vi "Length_7.vi"() -> ()   [LabVIEW 2020]
uses:
  Support/Controls/Cmd_Mouse Popup.ctl
  Support/Controls/Clst_Initialize Input.ctl
  Support/Controls/Cmd_Var Data IO.ctl
  Variables/Global_Cal Info.vi
  Variables/Global_Cal STD.vi
  Support/Public/Polymorph/Data Class_2D Str.vi
panel:
  out "STD set":string[][](table) caption="○ 기준기 조합 (값)"
  in  "기준기 설정":string(combo)
  in  "Measured 3":string[][](table)
  in  "Measured 2":string[][](table) caption="평행도 (μm)"
  out "최소범위":string
  out "단위":string
  out "최대범위":string
  in  "Spec 변경":bool
  in  "Random":bool
  out "Spec":string[][](table)
  out "제목":string
  out "에러 출력":errorcluster
  out "Condition":string[][](table) caption="2. 직선성 시험"
  in  "Measured":string[][](table) caption="지시편차 (μm)"
  out "Load?":bool
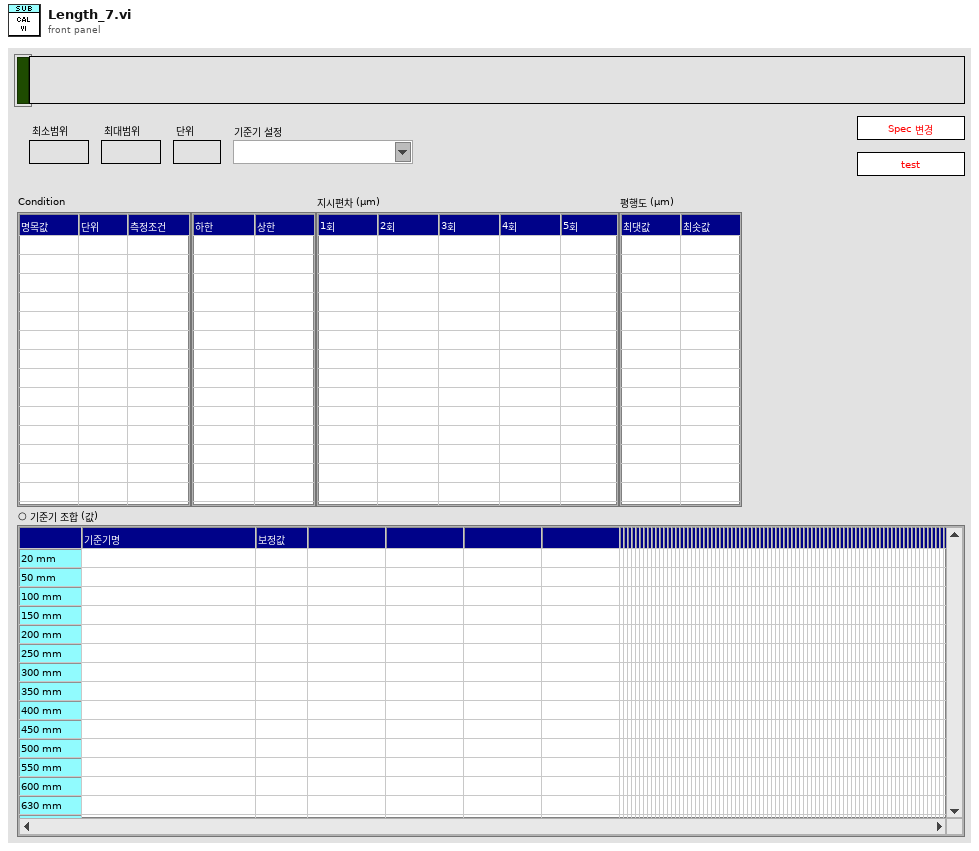
[diagram p1: front panel]
types:
  T1 = typedef "Cmd_Mouse Popup.ctl" = enum16{"활성화", "메뉴선택"}
  T2 = cluster{"Shift":bool, "Ctrl":bool, "Alt":bool, "Cmd":bool, "Opt":bool}
  T3 = typedef "Clst_Initialize Input.ctl" = cluster{"Initialize 1":cluster{"Condition":refnum<vi>[], "Spec":refnum<vi>[], "Measured":refnum<vi>[], "Resolution":refnum<vi>[], "Func_ext":string, "제목":refnum<vi>, "Measured_ADJ":refnum<vi>[]}, "Initialize 2":cluster{"문자열":refnum<vi>[], "콤보박스":refnum<vi>[], "링":refnum<vi>[], "열거형":refnum<vi>[], "테이블":refnum<vi>[], "여러열":refnum<vi>[], "디지털(DBL)":refnum<vi>[], "3D string":refnum<vi>[], "ctrl":refnum<vi>[], "boolean":refnum<vi>[]}}
  T4 = typedef "Cmd_Var Data IO.ctl" = enum16{"Condition", "Condition Default", "Condition_Temp", "Resolution", "Resolution Default", "Resolution Old", "Spec", "Spec Default", "Spec Old", "Spec Temp", "Result", "Result2", "Result3", "Result_Temp", "Result_ADJ", "Result_ADJ2", "STD1", "STD2", "STD3", "STD4", "STD5", "STD Temp", "CMC", "CMC Default"}
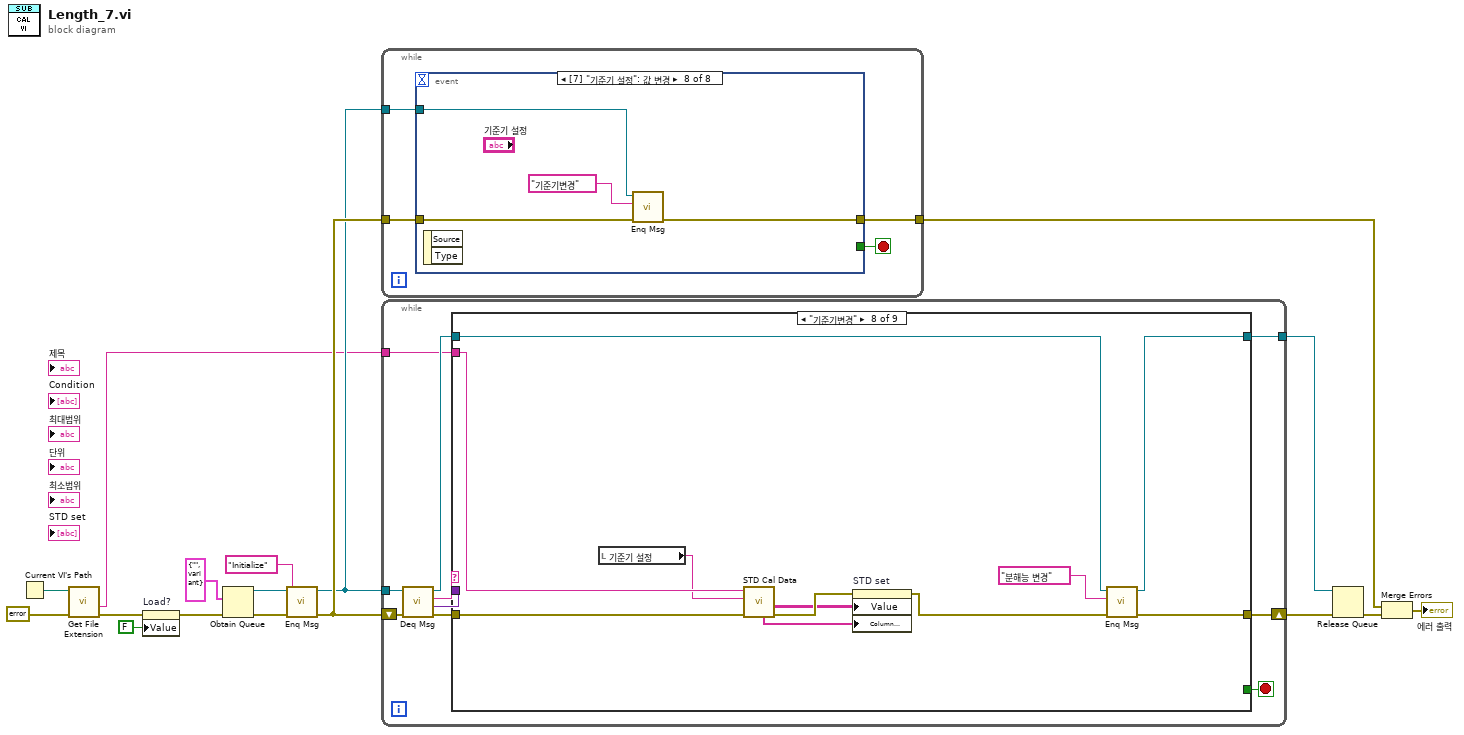
[diagram p0: block diagram]
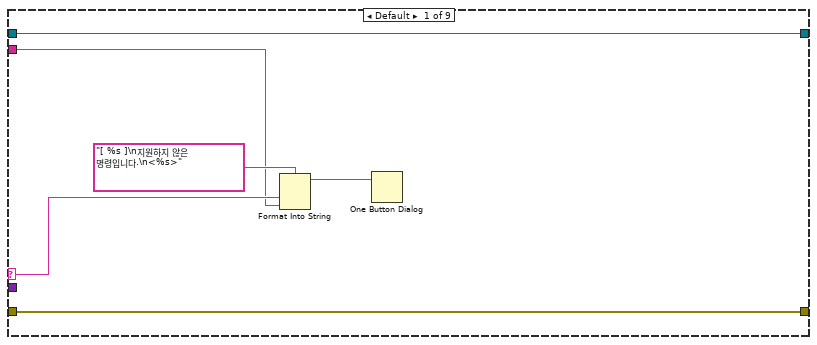
[diagram p2: hidden frame]
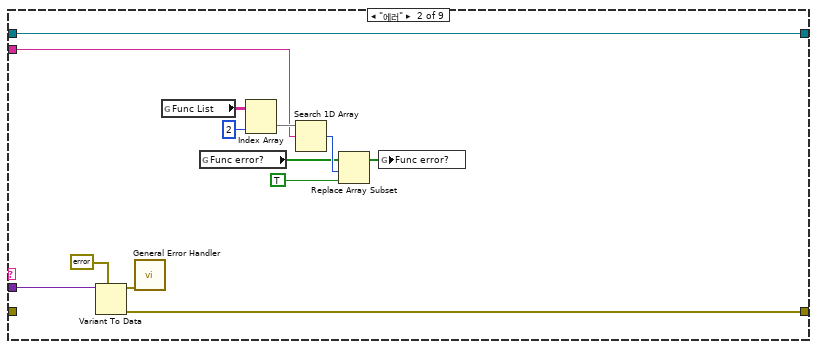
[diagram p3: hidden frame]
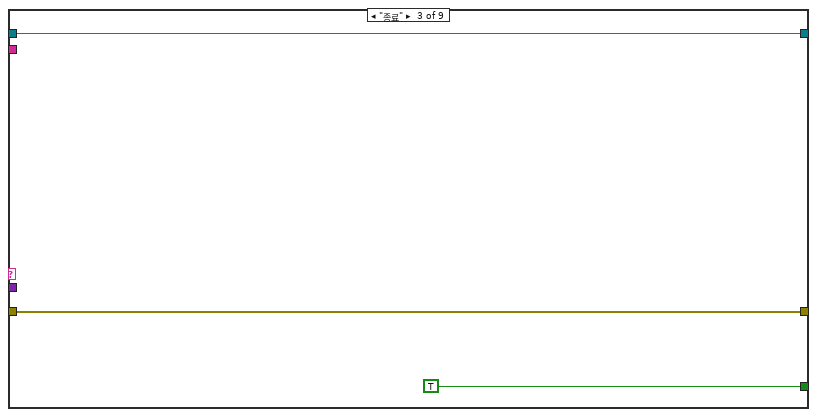
[diagram p4: hidden frame]
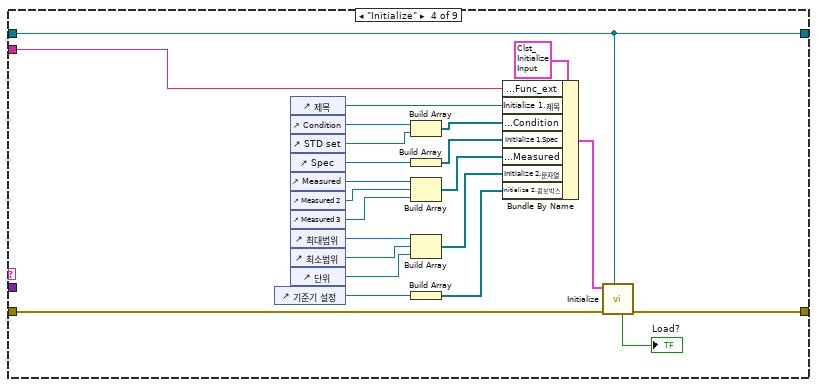
[diagram p5: hidden frame]
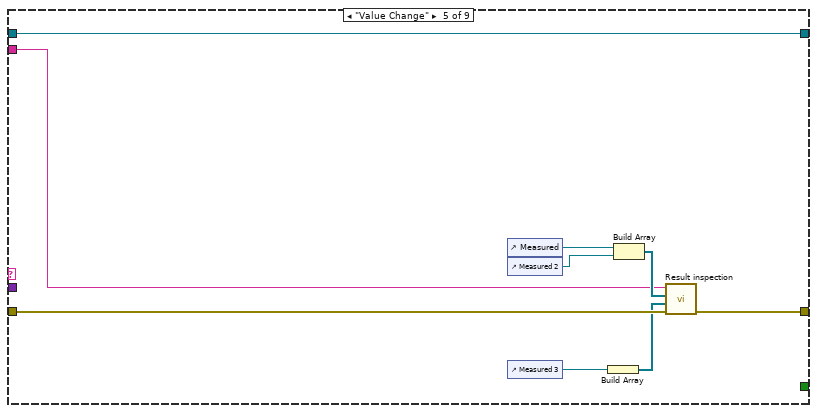
[diagram p6: hidden frame]
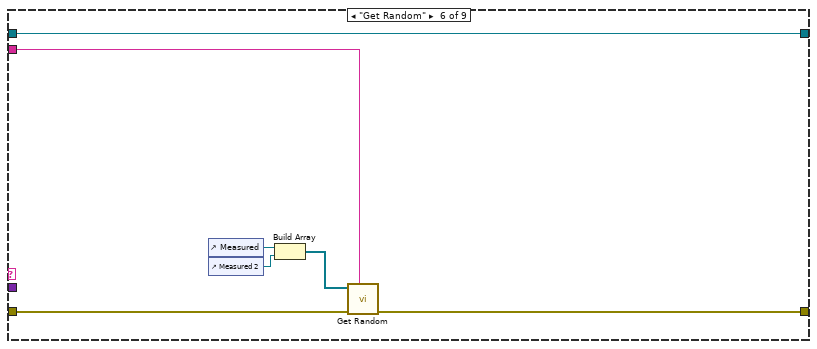
[diagram p7: hidden frame]
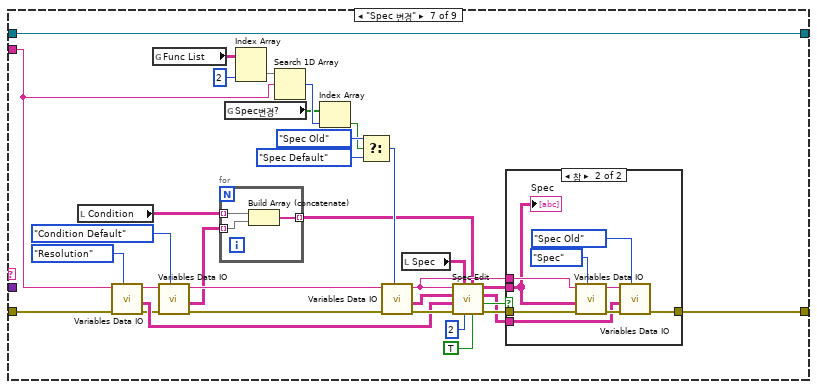
[diagram p8: hidden frame]
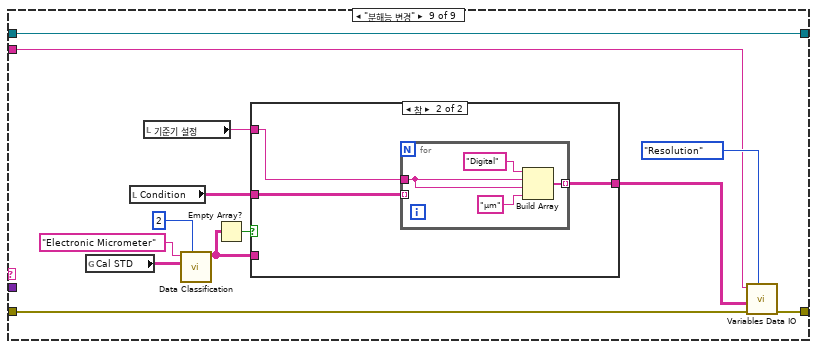
[diagram p10: hidden frame]
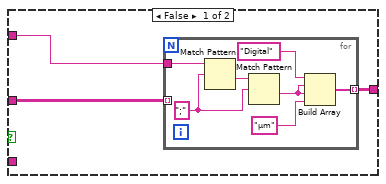
[diagram p11: hidden frame]
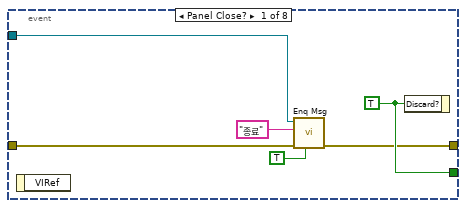
[diagram p12: hidden frame]
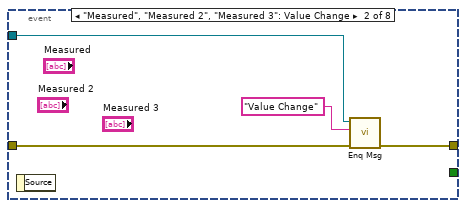
[diagram p13: hidden frame]
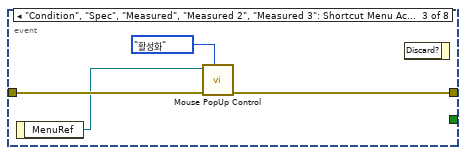
[diagram p14: hidden frame]
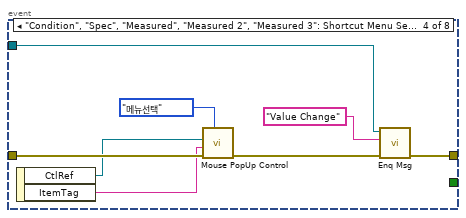
[diagram p15: hidden frame]
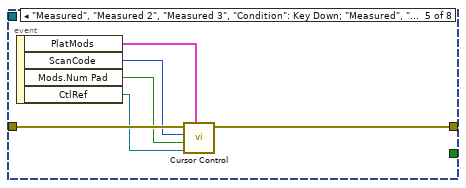
[diagram p16: hidden frame]
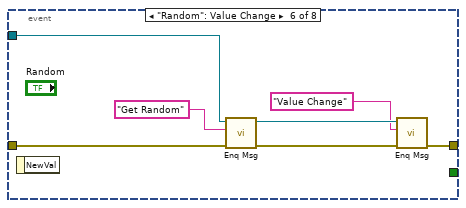
[diagram p17: hidden frame]
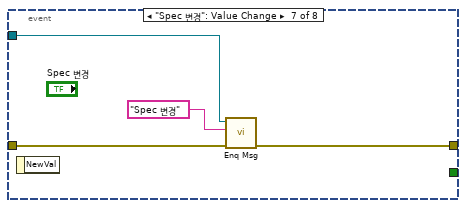
[diagram p18: hidden frame]
diagram:
  n1 = Current VI's Path() -> (path=w5:path)
  n2 = call <vilib>:"Get File Extension.vi"("error in (no error)"=errorcluster {"status"=FALSE, "code"=0, "source"=""} ("에러 상수"), "file"=w5) -> ("error out"=w3:errorcluster, "filename without extension"=w4:string)  [unwired: 5 in, 3 out]
  n3 = property on="Load?" class="Bool (엄격한)"(error in=w3, "Value"=FALSE ("Load?")) -> (error out=w2:errorcluster)  [unwired: 1 in, 1 out]
  n4 = Obtain Queue(element data type=cluster{"메세지":string, "값":variant} {"메세지"="", "값"=variant} ("Message Cluster"), error in (no error)=w2) -> (queue out=w14:refnum<queue>, error out=w16:errorcluster)  [unwired: 3 in, 1 out]
  n5 = call "Enq Msg.vi"("에러 입력(에러 없음)"=w16, "메세지"="Initialize", "큐 입력"=w14) -> ("에러 출력"=w15:errorcluster, "큐 출력"=w12:refnum<queue>)  [unwired: 7 in]
  n6 = while {
    tunnel: w15 -> [w19]
    tunnel: w12 -> [w20]
    tunnel: [w18] -> w9
    stop <- w21 stop-if-true
    n7 = event shown="[7] \"기준기 설정\": 값 변경" {
      selector: _ -> [_ _ _ _ _ _ _ _]
      dyn-events: _ -> [_ _ _ _ _ _ _ _]
      timeout: _ -> [_ _ _ _ _ _ _ _]
      tunnel: [w27 _ _ _ _ _ _ _] -> w21
      tunnel: w20 -> [w25 w31 _ w36 _ w54 w58 w62]
      tunnel: w19 -> [w26 w29 w35 w43 w49 w55 w59 w63]
      tunnel: [w23 w30 w34 w37 w48 w50 w57 w61] -> w18
      event Panel Close? {
        w27 = TRUE ("버림?")
        n8 = event-data() -> ()  [unwired: 1 in, 1 out]
        n9 = call "Enq Msg.vi"("우선순위 메시지?"=TRUE, "에러 입력(에러 없음)"=w26, "메세지"="종료", "큐 입력"=w25) -> ("에러 출력"=w23:errorcluster)  [unwired: 6 in, 1 out]
        n10 = event-data("Discard?"=w27) -> ()  [unwired: 1 in, 1 out]
      }
      event "Measured", "Measured 2", "Measured 3": Value Change {
        n11 = event-data() -> ()  [unwired: 1 in, 1 out]
        n12 = call "Enq Msg.vi"("에러 입력(에러 없음)"=w29, "메세지"="Value Change", "큐 입력"=w31) -> ("에러 출력"=w30:errorcluster)  [unwired: 7 in, 1 out]
      }
      event "Condition", "Spec", "Measured", "Measured 2", "Measured 3": Shortcut Menu Activation? {
        n13 = event-data() -> ("MenuRef"=w33:refnum<k9>)  [unwired: 1 in]
        n14 = call "Mouse PopUp Control.vi"("type"=Cmd_Mouse_Popup."활성화", "error in"=w35, "메뉴 참조"=w33) -> ("error out"=w34:errorcluster)  [unwired: 8 in]
        n15 = event-data() -> ()  [unwired: 2 in, 1 out]
      }
      event "Condition", "Spec", "Measured", "Measured 2", "Measured 3": Shortcut Menu Selection (User) {
        n16 = event-data() -> ("CtlRef"=w41:refnum<vi>, "ItemTag"=w40:string)  [unwired: 1 in]
        n17 = call "Mouse PopUp Control.vi"("type"=Cmd_Mouse_Popup."메뉴선택", "error in"=w43, "아이템 태그"=w40, "Tbl 참조 번호"=w41) -> ("error out"=w38:errorcluster)  [unwired: 7 in]
        n18 = call "Enq Msg.vi"("에러 입력(에러 없음)"=w38, "메세지"="Value Change", "큐 입력"=w36) -> ("에러 출력"=w37:errorcluster)  [unwired: 7 in, 1 out]
      }
      event "Measured", "Measured 2", "Measured 3", "Condition": Key Down; "Measured", "Measured 2", "Measured 3", "Condition": Key Repeat {
        n19 = event-data() -> ("PlatMods"=w44:T2, "ScanCode"=w47:i16, "Mods.Num Pad"=w46:bool, "CtlRef"=w45:refnum<vi>)  [unwired: 1 in]
        n20 = call "Cursor Control.vi"("플랫폼 조합키"=w44, "참조"=w45, "Num Pad"=w46, "ScanCode"=w47, "error in"=w49) -> ("error out"=w48:errorcluster)  [unwired: 5 in, 1 out]
      }
      event "Random": Value Change {
        n21 = event-data() -> ()  [unwired: 1 in, 1 out]
        n22 = call "Enq Msg.vi"("에러 입력(에러 없음)"=w55, "메세지"="Get Random", "큐 입력"=w54) -> ("에러 출력"=w53:errorcluster, "큐 출력"=w52:refnum<queue>)  [unwired: 7 in]
        n23 = call "Enq Msg.vi"("에러 입력(에러 없음)"=w53, "메세지"="Value Change", "큐 입력"=w52) -> ("에러 출력"=w50:errorcluster)  [unwired: 7 in, 1 out]
      }
      event "Spec 변경": Value Change {
        n24 = event-data() -> ()  [unwired: 1 in, 1 out]
        n25 = call "Enq Msg.vi"("에러 입력(에러 없음)"=w59, "메세지"="Spec 변경", "큐 입력"=w58) -> ("에러 출력"=w57:errorcluster)  [unwired: 7 in, 1 out]
      }
      event "기준기 설정": Value Change {
        n26 = event-data() -> ()  [unwired: 1 in, 2 out]
        n27 = call "Enq Msg.vi"("에러 입력(에러 없음)"=w63, "메세지"="기준기변경", "큐 입력"=w62) -> ("에러 출력"=w61:errorcluster)  [unwired: 7 in, 1 out]
      }
    }
  }
  n28 = while {
    shift-right: [w74] -> w11
    shift-left: w15 -> [w73]
    tunnel: w12 -> [w71]
    tunnel: [w66] -> w10
    tunnel: w4 -> [w65]
    stop <- w67 stop-if-true
    n29 = call "Deq Msg.vi"("에러 입력(에러 없음)"=w73, "큐 입력"=w71) -> ("에러 출력"=w72:errorcluster, "값"=w68:variant, "메세지"=w70:string, "큐 출력"=w69:refnum<queue>)  [unwired: 6 in]
    n30 = case shown="\"기준기변경\"" w70 {
      selector: w70 -> [w76 _ _ _ _ _ _ _ _]
      tunnel: w72 -> [w80 _ w96 w119 w124 w131 w161 w192 w194]
      tunnel: [w80 w90 w96 w111 w127 w132 w164 w184 w202] -> w74
      tunnel: w69 -> [w79 w89 w94 w107 w128 w135 w168 w183 w205]
      tunnel: w68 -> [_ w91 _ _ _ _ _ _ _]
      tunnel: [_ _ TRUE ("버림?") _ _ _ _ _ _] -> w67
      tunnel: [w79 w89 w94 w107 w128 w135 w168 w182 w205] -> w66
      tunnel: w65 -> [w75 w81 _ w108 w123 w130 w146 w191 w193]
      frame Default {
        n31 = Format Into String(format string="[ %s ]\n지원하지 않은 명령입니다.\n<%s>" ("메시지"), w76, w75) -> (resulting string=w77:string)  [unwired: 2 in, 1 out]
        n32 = One Button Dialog(message=w77) -> ()  [unwired: 1 in, 1 out]
      }
      frame "에러" {
        n33 = Variant To Data(type=errorcluster {"status"=FALSE, "code"=0, "source"=""} ("에러 출력"), Variant=w91) -> (data=w93:errorcluster, error out=w90:errorcluster)  [unwired: 1 in]
        n34 = call <vilib>:"General Error Handler.vi"("error in (no error)"=w93) -> ()  [unwired: 10 in, 5 out]
        n35 = global read "Global_Cal Info.vi" "Func List"() -> (w83:string[][])
        n36 = global read "Global_Cal Info.vi" "Func error?"() -> (w86:bool[])
        n37 = Index Array(array=w83, index (col)=2 ("비활성화된 인덱스 (열)")) -> (element=w84:string[])  [unwired: 1 in]
        n38 = Search 1D Array(1D array=w84, element=w81) -> (index of element=w87:i32)  [unwired: 1 in]
        n39 = Replace Array Subset(array=w86, new element=TRUE ("새 원소/부분배열"), index=w87) -> (w88:bool[])
        n40 = global write "Global_Cal Info.vi" "Func error?"(w88) -> ()
      }
      frame "종료" {
      }
      frame "Initialize" {
        n41 = control-ref of="기준기 설정"() -> (w101:refnum<vi>)
        n42 = control-ref of="제목"() -> (w112:refnum<vi>)
        n43 = control-ref of="Condition"() -> (w116:refnum<vi>)
        n44 = control-ref of="STD set"() -> (w99:refnum<vi>)
        n45 = control-ref of="Spec"() -> (w110:refnum<vi>)
        n46 = control-ref of="Measured"() -> (w113:refnum<vi>)
        n47 = control-ref of="Measured 2"() -> (w102:refnum<vi>)
        n48 = control-ref of="Measured 3"() -> (w98:refnum<vi>)
        n49 = control-ref of="최대범위"() -> (w103:refnum<vi>)
        n50 = control-ref of="최소범위"() -> (w104:refnum<vi>)
        n51 = control-ref of="단위"() -> (w106:refnum<vi>)
        n52 = Build Array(w116, w99) -> (w115:refnum<vi>[])
        n53 = Build Array(w110) -> (w109:refnum<vi>[])
        n54 = Build Array(w113, w102, w98) -> (w114:refnum<vi>[])
        n55 = Build Array(w103, w104, w106) -> (w105:refnum<vi>[])
        n56 = Build Array(w101) -> (w100:refnum<vi>[])
        n57 = Bundle By Name(cluster=T3 {"Initialize 1"={"Condition"=[], "Spec"=[], "Measured"=[], "Resolution"=[], "Func_ext"="", "제목"=refnum, "Measured_ADJ"=[]}, "Initialize 2"={"문자열"=[], "콤보박스"=[], "링"=[], "열거형"=[], "테이블"=[], "여러열"=[], "디지털(DBL)"=[], "3D string"=[], "ctrl"=[], "boolean"=[]}} ("입력 클러스터"), "Initialize 1.Func_ext"=w108, "Initialize 1.제목"=w112, "Initialize 1.Condition"=w115, "Initialize 1.Spec"=w109, "Initialize 1.Measured"=w114, "Initialize 2.문자열"=w105, "Initialize 2.콤보박스"=w100) -> (w117:T3)
        n58 = call "Initialize.vi"("큐 입력"=w107, "error in"=w119, "입력 클러스터"=w117) -> ("error out"=w111:errorcluster, "Load?"=→"Load?":bool)  [unwired: 5 in, 2 out]
      }
      frame "Value Change" {
        n59 = control-ref of="Measured"() -> (w126:refnum<vi>)
        n60 = control-ref of="Measured 2"() -> (w120:refnum<vi>)
        n61 = control-ref of="Measured 3"() -> (w121:refnum<vi>)
        n62 = Build Array(w121) -> (w122:refnum<vi>[])
        n63 = Build Array(w126, w120) -> (w125:refnum<vi>[])
        n64 = call "Result inspection.vi"("error in"=w124, "Ref. Data (excluded)"=w122, "Ref. Data (Inspection)"=w125, "Func ext"=w123) -> ("error out"=w127:errorcluster)  [unwired: 4 in, 3 out]
      }
      frame "Get Random" {
        n65 = control-ref of="Measured"() -> (w134:refnum<vi>)
        n66 = control-ref of="Measured 2"() -> (w129:refnum<vi>)
        n67 = Build Array(w134, w129) -> (w133:refnum<vi>[])
        n68 = call "Get Random.vi"("Func_Ext"=w130, "에러 입력"=w131, "Meas"=w133) -> ("에러 출력"=w132:errorcluster)  [unwired: 7 in, 1 out]
      }
      frame "Spec 변경" {
        n69 = local read "Condition"() -> (w139:string[][])
        n70 = call "Variables Data IO.vi"("Select"=Cmd_Var_Data_IO."Resolution", "error in"=w161, "Func_ext"=w146) -> ("error out"=w144:errorcluster, "Data Out"=w155:string[][], "Func_ext Out"=w142:string)  [unwired: 6 in]
        n71 = global read "Global_Cal Info.vi" "Func List"() -> (w151:string[][])
        n72 = call "Variables Data IO.vi"("Select"=Cmd_Var_Data_IO."Condition Default", "error in"=w144, "Func_ext"=w142) -> ("error out"=w143:errorcluster, "Data Out"=w138:string[][], "Func_ext Out"=w141:string)  [unwired: 6 in]
        n73 = for {
          tunnel: w139 -> [w171] mode=indexing
          tunnel: w138 -> [w170] mode=indexing
          tunnel: [w169] -> w137 mode=indexing
          n74 = Build Array (concatenate)(w171, w170) -> (w169:string[])
        }
        n75 = global read "Global_Cal Info.vi" "Spec변경?"() -> (w147:bool[])
        n76 = Index Array(array=w151, index (col)=2 ("비활성화된 인덱스 (열)")) -> (element=w149:string[])  [unwired: 1 in]
        n77 = Search 1D Array(1D array=w149, element=w146) -> (index of element=w148:i32)  [unwired: 1 in]
        n78 = Index Array(array=w147, index=w148) -> (element=w152:bool)
        n79 = Select(t=Cmd_Var_Data_IO."Spec Old" ("Select"), s=w152, f=Cmd_Var_Data_IO."Spec Default" ("Select")) -> (s? t:f=w145:T4)
        n80 = call "Variables Data IO.vi"("Select"=w145, "error in"=w143, "Func_ext"=w141) -> ("error out"=w163:errorcluster, "Data Out"=w156:string[][], "Func_ext Out"=w157:string)  [unwired: 6 in]
        n81 = local read "Spec"() -> (w158:string[][])
        n82 = call "Spec Edit.vi"("0기준?"=TRUE, "Condition"=w137, "열번호(기준값)"=2, "Spec Value"=w158, "에러 입력(에러 없음)"=w163, "Resolution"=w155, "Spec Default"=w156, "Func_ext"=w157) -> ("에러 출력"=w165:errorcluster, "변경?"=w166:bool, "Spec Default out"=w160:string[][], "Spec 출력"=w167:string[][])
        n83 = case shown="참" w166 {
          tunnel: w167 -> [_ w178]
          tunnel: w165 -> [w172 w181]
          tunnel: [w172 w176] -> w164
          tunnel: w157 -> [_ w179]
          tunnel: w160 -> [_ w174]
          frame False {
          }
          frame True {
            n84 = call "Variables Data IO.vi"("Select"=Cmd_Var_Data_IO."Spec", "error in"=w181, "Data In"=w178, "Func_ext"=w179) -> ("error out"=w177:errorcluster, "Func_ext Out"=w175:string)  [unwired: 5 in, 1 out]
            n85 = call "Variables Data IO.vi"("Select"=Cmd_Var_Data_IO."Spec Old", "error in"=w177, "Data In"=w174, "Func_ext"=w175) -> ("error out"=w176:errorcluster)  [unwired: 5 in, 2 out]
            "Spec" <- w178
          }
        }
      }
      frame "기준기변경" {
        n86 = local read "기준기 설정"() -> (w190:string)
        n87 = call "STD Cal Data.vi"("error in"=w192, "문자열"=w190, "Func_ext"=w191) -> ("error out"=w189:errorcluster, "Data Out"=w187:string[][], "Data Out 2"=w188:string[])  [unwired: 4 in, 2 out]
        n88 = property on="STD set" class="Tbl (엄격한)"(error in=w189, "Value"=w187, "Column Headers[]"=w188) -> (error out=w185:errorcluster)  [unwired: 1 in, 1 out]
        n89 = call "Enq Msg.vi"("에러 입력(에러 없음)"=w185, "메세지"="분해능 변경", "큐 입력"=w183) -> ("에러 출력"=w184:errorcluster, "큐 출력"=w182:refnum<queue>)  [unwired: 7 in]
      }
      frame "분해능 변경" {
        n90 = global read "Global_Cal STD.vi" "Cal STD"() -> (w198:string[][])
        n91 = local read "Condition"() -> (w195:string[][])
        n92 = local read "기준기 설정"() -> (w204:string)
        n93 = call-poly "Data Classification.vi"("인덱스"=2, "DATA 입력"=w198, "검색 문자열"="Electronic Micrometer") -> ("DATA 출력"=w197:string[][])  [unwired: 4 in, 4 out]
        n94 = Empty Array?(array=w197) -> (empty?=w196:bool)
        n95 = case shown="참" w196 {
          tunnel: w204 -> [w208 w218]
          tunnel: [w207 w217] -> w201
          tunnel: w197 -> [_ _]
          tunnel: w195 -> [w206 w216]
          frame False {
            n96 = for {
              tunnel: w208 -> [w210]
              tunnel: [w215] -> w207 mode=indexing
              tunnel: w206 -> [_] mode=indexing
              w211 = ";" ("정규식")
              n97 = Match Pattern(string=w210, regular expression=w211) -> (after substring=w212:string)  [unwired: 1 in, 3 out]
              n98 = Match Pattern(string=w212, regular expression=w211) -> (after substring=w209:string)  [unwired: 1 in, 3 out]
              n99 = Build Array("Digital" ("원소"), w209, w209, "μm" ("원소")) -> (w215:string[])
            }
          }
          frame True {
            n100 = for {
              tunnel: w218 -> [w219]
              tunnel: [w222] -> w217 mode=indexing
              tunnel: w216 -> [_] mode=indexing
              n101 = Build Array("Digital" ("원소"), w219, w219, "μm" ("원소")) -> (w222:string[])
            }
          }
        }
        n102 = call "Variables Data IO.vi"("Select"=Cmd_Var_Data_IO."Resolution", "error in"=w194, "Data In"=w201, "Func_ext"=w193) -> ("error out"=w202:errorcluster)  [unwired: 5 in, 2 out]
      }
    }
  }
  n103 = Release Queue(queue=w10, error in (no error)=w11) -> (error out=w8:errorcluster)  [unwired: 1 in, 2 out]
  n104 = Merge Errors(w9, w8) -> (→"에러 출력":errorcluster)
